vi "평균 및 숫자 출력 예제.vi"() -> ()   [LabVIEW 2025]
panel:
  out "length":i32
  out "String":string
  in  "과학 2":dbl
  in  "수학":dbl
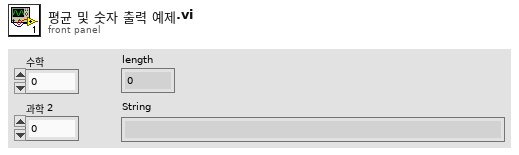
[diagram p1: front panel]
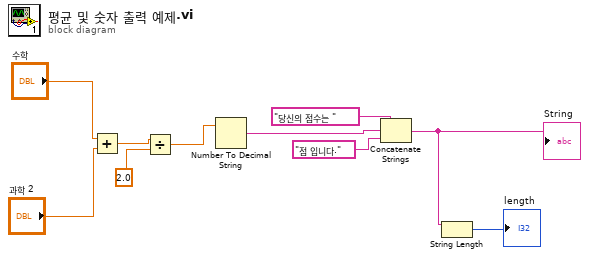
[diagram p0: block diagram]
diagram:
  n1 = Add(x="수학", y="과학 2") -> (x+y=w8:dbl)
  n2 = Divide(x=w8, y=2.0) -> (x/y=w6:dbl)
  n3 = Number To Decimal String(number=w6) -> (decimal integer string=w4:string)  [unwired: 1 in]
  n4 = Concatenate Strings("당신의 점수는 " ("string"), w4, "점 입니다." ("string")) -> (w2:string)
  "String" <- w2
  n5 = String Length(string=w2) -> (length=→"length":i32)
